vi "Disconnect.vi"(8 "error in":errorcluster, 11 "PRM in":refnum<class "PRM.lvclass">) -> (0 "error out":errorcluster, 3 "PRM out":refnum<class "PRM.lvclass">)   [LabVIEW 2019, in "PRM.lvlib" / "PRM.lvclass"]
uses:
  Library/PRM.lvclass
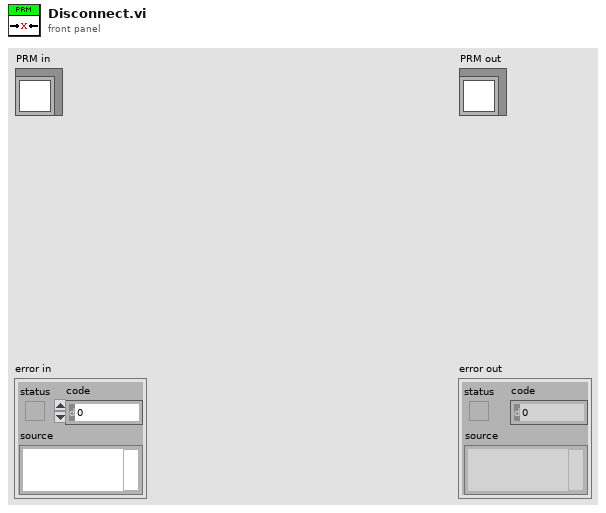
[diagram p1: front panel]
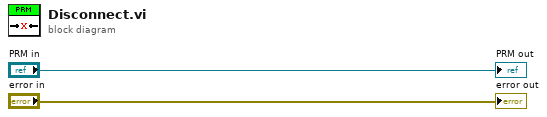
[diagram p0: block diagram]
diagram:
  "error out" <- "error in"
  "PRM out" <- "PRM in"
